vi "oa_Check Time-RPM Segments.vi"(0 "processing mode":u16(ring) items=["Continuous", "Compute at Time Interval", "Compute at Speed Interval"], 1 "reset?(F)":bool, 5 "Limit range":bool, 7 "steps input":cluster{"start":dbl, "end":dbl, "step":dbl} {"step" format="%.2f"; "end" format="%.2f"; "start" format="%.2f"}, 9 "speed profile":T1 {"speed [RPM]" format="%.2f"; "time [s]" format="%.2f"}, 11 "error in (no error)":errorcluster) -> (4 "processing mode duplicate":u16, 6 "step found?":bool, 8 "steps output":cluster{"start":dbl, "end":dbl, "step":dbl}, 10 "speed profile duplicate":T1 {"speed [RPM]" format="%.2f"; "time [s]" format="%.2f"}, 15 "error out":errorcluster)   [LabVIEW 2017, in "SoundVib_OAUtility.lvlib"]
uses:
  <vilib>/addons/Sound and Vibration/Order Analysis/Utility/SoundVib_OAUtility.lvlib
  <vilib>/addons/Sound and Vibration/Order Analysis/Tach Process/SubVIs/speed profile.ctl
  <vilib>/addons/Sound and Vibration/Order Analysis/Tach Process/SoundVib_TachProcess.lvlib
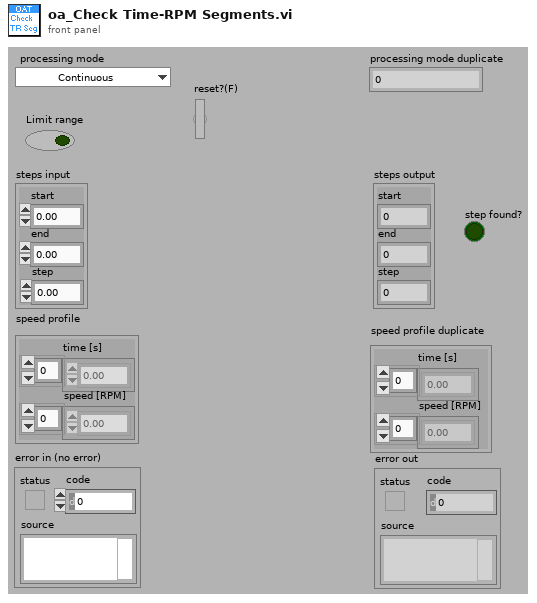
[diagram p1: front panel]
types:
  T1 = typedef "SoundVib_TachProcess.lvlib/speed profile.ctl" = cluster{"time [s]":dbl[], "speed [RPM]":dbl[]}
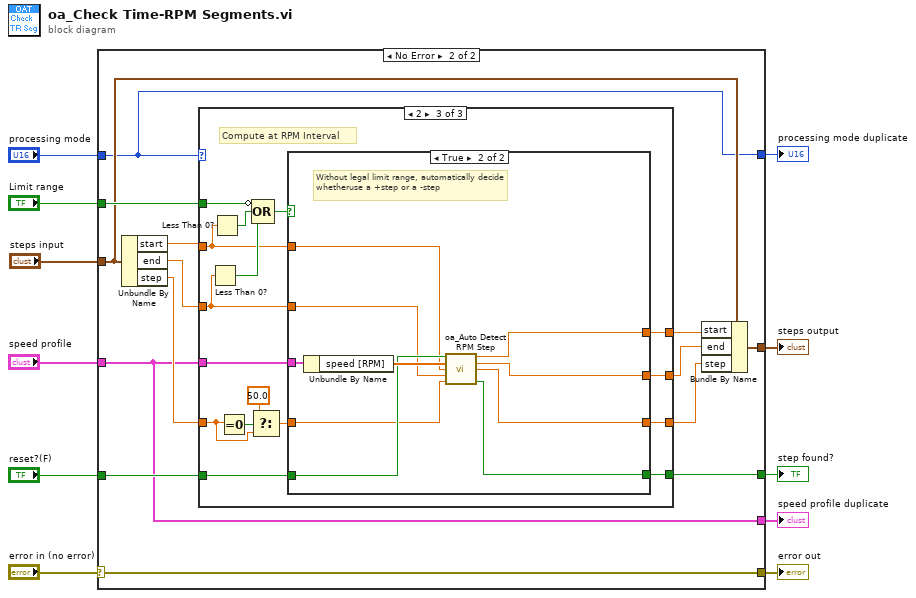
[diagram p0: block diagram]
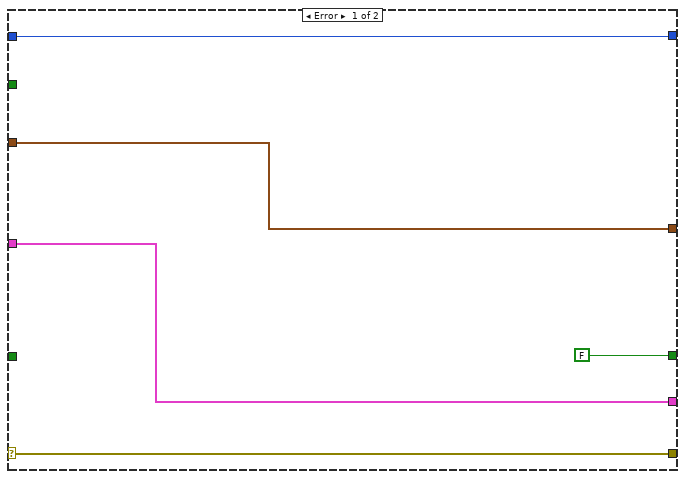
[diagram p2: hidden frame]
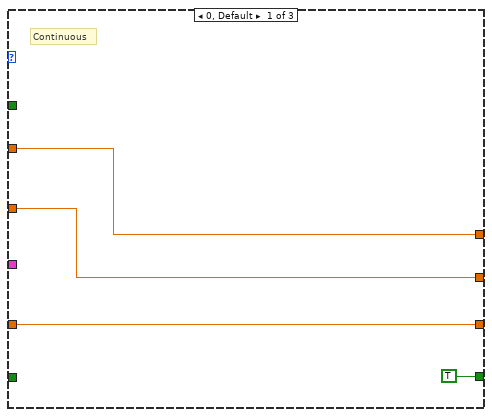
[diagram p3: hidden frame]
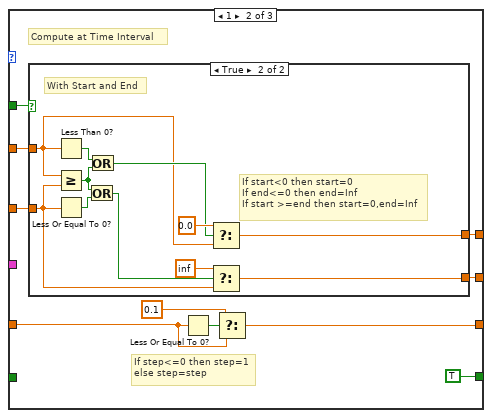
[diagram p4: hidden frame]
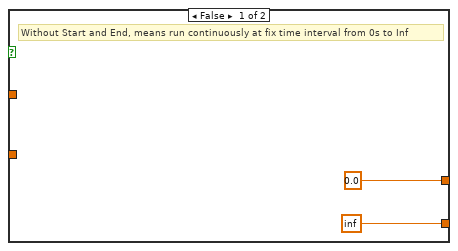
[diagram p5: hidden frame]
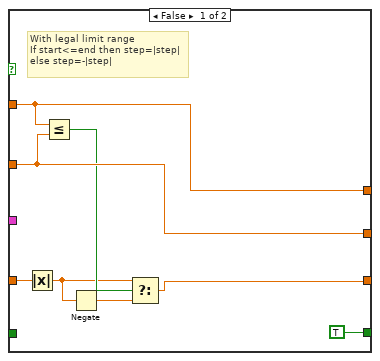
[diagram p6: hidden frame]
diagram:
  n1 = case shown="No Error" "error in (no error)" {
    selector: "error in (no error)" -> [w16 w29]
    tunnel: "processing mode" -> [w13 w18]
    tunnel: "steps input" -> [w14 w23]
    tunnel: "Limit range" -> [_ w30]
    tunnel: "speed profile" -> [w12 w17]
    tunnel: [w16 w29] -> w7
    tunnel: "reset?(F)" -> [_ w28]
    tunnel: [FALSE ("step found?") w27] -> w5
    tunnel: [w14 w19] -> w3
    tunnel: [w13 w18] -> w1
    tunnel: [w12 w17] -> w2
    frame Error {
    }
    frame No Error {
      n2 = Unbundle By Name(w23) -> ("start"=w26:dbl, "end"=w25:dbl, "step"=w24:dbl)
      n3 = case shown="2" w18 {
        tunnel: w26 -> [w32 w41 w68]
        tunnel: w25 -> [w33 w42 w67]
        tunnel: w24 -> [w34 w36 w60]
        tunnel: [w32 w44 w66] -> w22
        tunnel: [w33 w43 w65] -> w21
        tunnel: [w34 w35 w64] -> w20
        tunnel: w30 -> [_ w40 w73]
        tunnel: w17 -> [_ _ w69]
        tunnel: w28 -> [_ _ w63]
        tunnel: [TRUE ("step found?") TRUE ("step found?") w62] -> w27
        frame 0, Default {
          # "Continuous"
        }
        frame 1 {
          # "If step<=0 then step=1\nelse step=step"
          # "Compute at Time Interval"
          n4 = case shown="True" w40 {
            tunnel: [0.0 ("start input") w56] -> w44
            tunnel: [inf ("end input") w57] -> w43
            tunnel: w42 -> [_ w51]
            tunnel: w41 -> [_ w47]
            frame False {
              # "Without Start and End, means run continuously at fix time interval from 0s to Inf"
            }
            frame True {
              # "If start<0 then start=0\nIf end<=0 then end=Inf\nIf start >=end then start=0,end=Inf"
              # "With Start and End"
              n5 = Less Than 0?(x=w47) -> (x < 0?=w50:bool)
              n6 = Greater Or Equal?(x=w47, y=w51) -> (x >= y?=w49:bool)
              n7 = Less Or Equal To 0?(x=w51) -> (x <= 0?=w53:bool)
              n8 = Or(x=w49, y=w53) -> (x .or. y?=w52:bool)
              n9 = Or(x=w50, y=w49) -> (x .or. y?=w48:bool)
              n10 = Select(t=0.0, s=w48, f=w47) -> (s? t:f=w56:dbl)
              n11 = Select(t=inf ("f"), s=w52, f=w51) -> (s? t:f=w57:dbl)
            }
          }
          n12 = Less Or Equal To 0?(x=w36) -> (x <= 0?=w37:bool)
          n13 = Select(t=0.1, s=w37, f=w36) -> (s? t:f=w35:dbl)
        }
        frame 2 {
          # "Compute at RPM Interval"
          n14 = Less Than 0?(x=w67) -> (x < 0?=w71:bool)
          n15 = Less Than 0?(x=w68) -> (x < 0?=w72:bool)
          n16 = Equal To 0?(x=w60) -> (x = 0?=w61:bool)
          n17 = Select(t=50.0, s=w61, f=w60) -> (s? t:f=w59:dbl)
          n18 = Compound Arithmetic op=OR(invert w73, w72, w71) -> (w70:bool)
          n19 = case shown="True" w70 {
            tunnel: w69 -> [_ w91]
            tunnel: w68 -> [w81 w88]
            tunnel: w67 -> [w80 w87]
            tunnel: w59 -> [w78 w86]
            tunnel: [w81 w85] -> w66
            tunnel: [w80 w84] -> w65
            tunnel: [w75 w83] -> w64
            tunnel: w63 -> [_ w89]
            tunnel: [TRUE ("step found?") w82] -> w62
            frame False {
              # "With legal limit range\nIf start<=end then step=|step|\nelse step=-|step|"
              n20 = Absolute Value(x=w78) -> (abs(x)=w77:dbl)
              n21 = Less Or Equal?(x=w81, y=w80) -> (x <= y?=w79:bool)
              n22 = Negate(x=w77) -> (-x=w76:dbl)
              n23 = Select(t=w77, s=w79, f=w76) -> (s? t:f=w75:dbl)
            }
            frame True {
              # "Without legal limit range, automatically decide whetheruse a +step or a -step"
              n24 = Unbundle By Name(w91) -> ("speed [RPM]"=w90:dbl[])
              n25 = call <vilib>:"oa_Auto Detect RPM Step.vi"("reset?"=w89, "speed(RPM)"=w90, "start input"=w88, "end input"=w87, "step input"=w86) -> ("start output"=w85:dbl, "end output"=w84:dbl, "step output"=w83:dbl, "step found?"=w82:bool)  [unwired: 7 in]
            }
          }
        }
      }
      n26 = Bundle By Name(cluster=w23, "start"=w22, "end"=w21, "step"=w20) -> (w19:cluster{"start":dbl, "end":dbl, "step":dbl})
    }
  }
  "error out" <- w7
  "step found?" <- w5
  "steps output" <- w3
  "speed profile duplicate" <- w2
  "processing mode duplicate" <- w1
